vi "Deadreckon Test.vi"() -> ()   [LabVIEW 2009]
uses:
  Remote Control/Motor Command.ctl
panel:
  out "MC init":bool
  in  "MC VISA resource in":refnum<visa-resource-name>="COM1"
  in  "stop":bool
  in  "GO !":bool
  in  "Time":dbl
  in  "Motor Command":T1
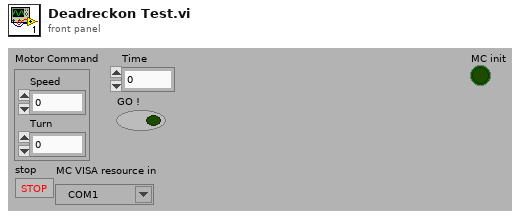
[diagram p1: front panel]
types:
  T1 = typedef "Motor Command.ctl" = cluster{"Speed":i16, "Turn":i16}
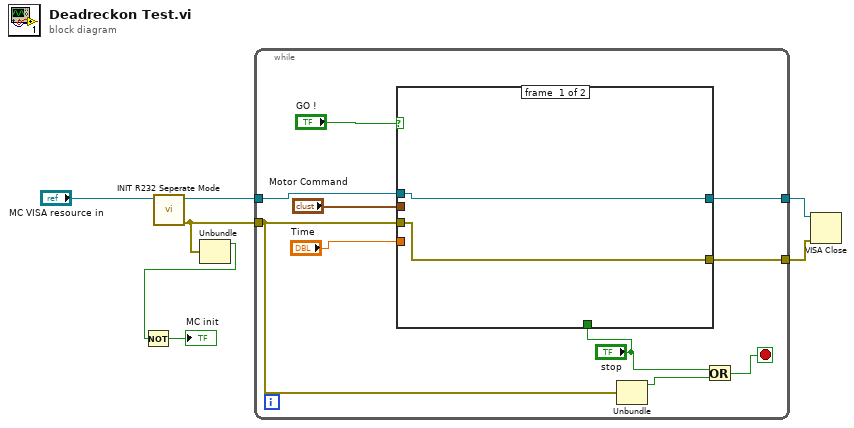
[diagram p0: block diagram]
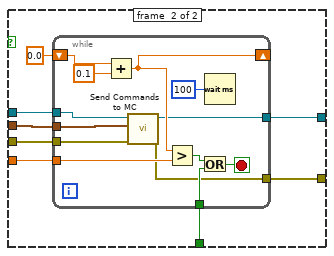
[diagram p2: hidden frame]
diagram:
  n1 = call "INIT R232 Seperate Mode.vi"("MC VISA resource in"="MC VISA resource in") -> ("MC error out"=w3:errorcluster, "MC VISA resource  out"=w7:refnum<visa-resource-name>)  [unwired: 8 in, 1 out]
  n2 = Unbundle(w3) -> ("status"=w2:bool)  [unwired: 2 out]
  n3 = Not(x=w2) -> (.not. x?=→"MC init":bool)
  n4 = while {
    tunnel: w7 -> [w14]
    tunnel: w3 -> [w9]
    tunnel: [w12] -> w6
    tunnel: [w13] -> w5
    stop <- w10 stop-if-true
    n5 = case shown="True" "GO !" {
      tunnel: "Motor Command" -> [_ w27]
      tunnel: "Time" -> [_ w26]
      tunnel: w14 -> [w19 w25]
      tunnel: w9 -> [w18 w24]
      tunnel: "stop" -> [_ w23]
      tunnel: [w19 w22] -> w12
      tunnel: [w18 w21] -> w13
      frame #0 {
      }
      frame #1 {
        n6 = while {
          tunnel: w27 -> [w40]
          tunnel: w26 -> [w38]
          shift-right: [w33] -> _
          shift-left: 0.0 -> [w36]
          tunnel: w25 -> [w32]
          tunnel: w24 -> [w31]
          tunnel: w23 -> [w30]
          tunnel: [w29] -> w22
          tunnel: [w28] -> w21
          stop <- w39 stop-if-true
          n7 = Add(x=w36, y=0.1) -> (x+y=w33:dbl)
          n8 = call "Send Commands to MC.vi"("MC refrence in"=w32, "Motor Command"=w40, "error in"=w31) -> ("MC refrence out"=w29:refnum<visa-resource-name>, "error out"=w28:errorcluster)  [unwired: 5 in, 1 out]
          n9 = Greater?(x=w33, y=w38) -> (0:w37:bool)
          n10 = Or(x=w37, y=w30) -> (x .or. y?=w39:bool)
          n11 = Wait (ms)(milliseconds to wait=u32 100) -> ()  [unwired: 1 out]
        }
      }
    }
    n12 = Unbundle(w9) -> ("status"=w8:bool)  [unwired: 2 out]
    n13 = Or(x="stop", y=w8) -> (x .or. y?=w10:bool)
  }
  n14 = VISA Close(VISA resource name=w6, error in (no error)=w5) -> ()  [unwired: 1 out]
